vi "Get Location Info.vi"(4 "Sand Grid":set{cdb}(c389), 5 "Rock Grid":set{cdb}(c389), 6 "Location":cdb, 9 "Grid Bounds":T1) -> (0 "Within the Grid ?":bool, 2 "Filled with Rock ?":bool, 3 "Filled with Sand ?":bool)   [LabVIEW 2020, in "AoC 2022.lvlib"]
uses:
  AoC 2022.lvlib
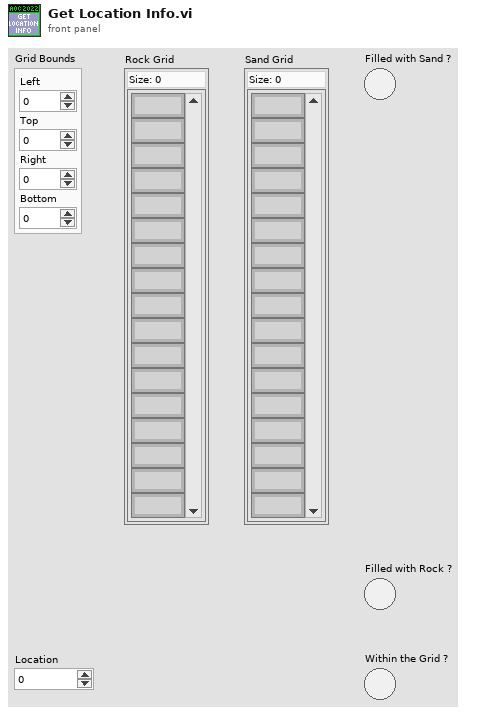
[diagram p1: front panel]
types:
  T1 = cluster{"Left":i16, "Top":i16, "Right":i16, "Bottom":i16}
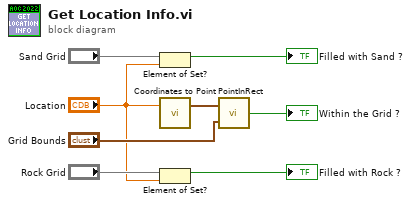
[diagram p0: block diagram]
diagram:
  n1 = Element of Set?(10:"Location", 11:"Sand Grid") -> (3:→"Filled with Sand ?":bool)
  n2 = call "Coordinates to Point.vi"("Coordinates"="Location") -> ("point"=w4:cluster{"x":dbl, "y":dbl})  [unwired: 2 in]
  n3 = Element of Set?(10:"Location", 11:"Rock Grid") -> (3:→"Filled with Rock ?":bool)
  n4 = call <vilib>:"PointInRect.vi"("rect"="Grid Bounds", "point"=w4) -> ("pt in rect"=→"Within the Grid ?":bool)
